vi "sensitivity_read.vi"(8 "error in (no error)":errorcluster, 11 "spectrIdx":u16) -> (0 "error out":errorcluster, 3 "sensitivity":u16)   [LabVIEW 2010, in "OSA.lvclass"]
uses:
  OSA.lvclass
  typeDef/sensitivityMode.ctl
  FTSLib.dll
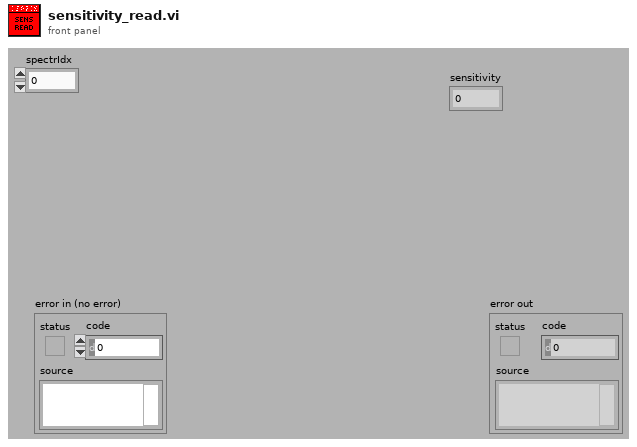
[diagram p1: front panel]
types:
  T1 = typedef "OSA.lvclass/sensitivityMode.ctl" = u16
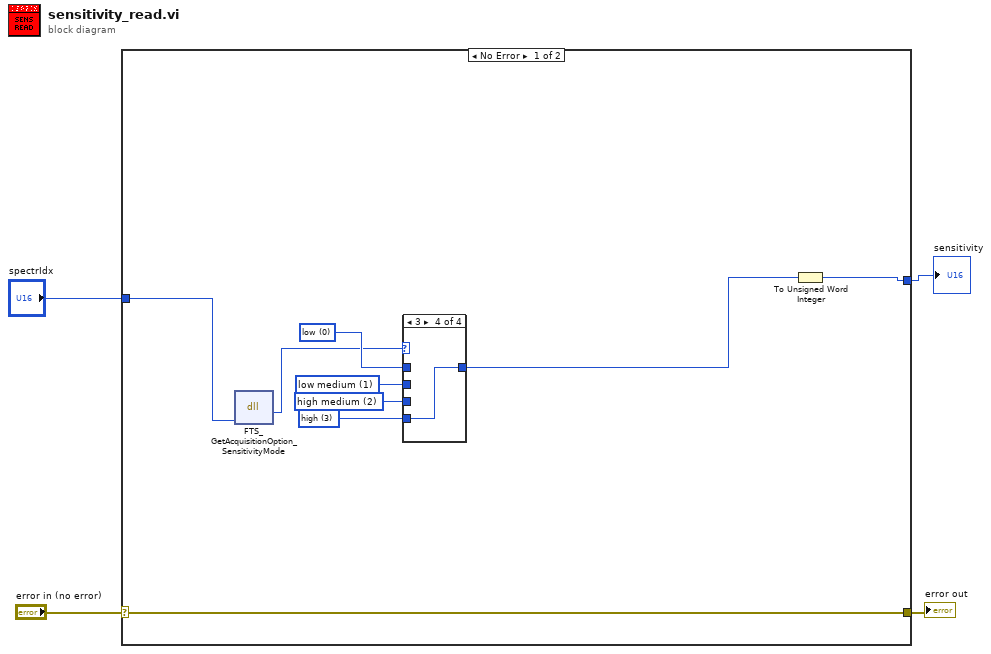
[diagram p0: block diagram]
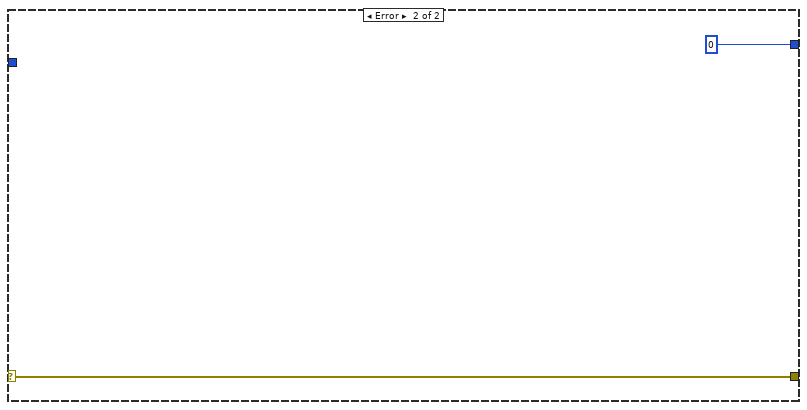
[diagram p5: hidden frame]
diagram:
  n1 = case shown="No Error" "error in (no error)" {
    selector: "error in (no error)" -> [w13 w19]
    tunnel: [w13 w19] -> w3
    tunnel: "spectrIdx" -> [w7 _]
    tunnel: [w5 u16 0] -> w1
    frame No Error {
      w9 = T1 0 items=["low", "low medium", "high medium", "high"] ("sensitivity")
      w10 = T1 1 items=["low", "low medium", "high medium", "high"] ("sensitivity")
      w11 = T1 2 items=["low", "low medium", "high medium", "high"] ("sensitivity")
      w12 = T1 3 items=["low", "low medium", "high medium", "high"] ("sensitivity")
      n2 = dll-call lib="FTSLib.dll" fn="FTS_GetAcquisitionOption_SensitivityMode"("spectrIdx"=w7) -> ("return type"=w8:i32)  [unwired: 4 in, 2 out]
      n3 = case shown="3" w8 {
        tunnel: [w14 w15 w16 w17] -> w6
        tunnel: w9 -> [_ w15 _ _]
        tunnel: w10 -> [w14 _ _ _]
        tunnel: w11 -> [_ _ w16 _]
        tunnel: w12 -> [_ _ _ w17]
        frame 0, Default {
        }
        frame 1 {
        }
        frame 2 {
        }
        frame 3 {
        }
      }
      n4 = To Unsigned Word Integer(number=w6) -> (unsigned 16bit integer=w5:T1)
    }
    frame Error {
    }
  }
  "error out" <- w3
  "sensitivity" <- w1
